vi "Special Folder Path.vi"(8 "error in (no error)":errorcluster, 11 "Special Folder":T1) -> (0 "error out":errorcluster, 3 "Path":path)   [LabVIEW 2013]
doc: "Return the path of the specified special folder. Calls SHGetFolderPathA routine in shell32.dll to determine the answer.\n\nFreeware from Moore Good Ideas, www.mooregoodideas.com. Do not remove this line."
uses:
  Special Folder Enum.ctl
  shell32.dll
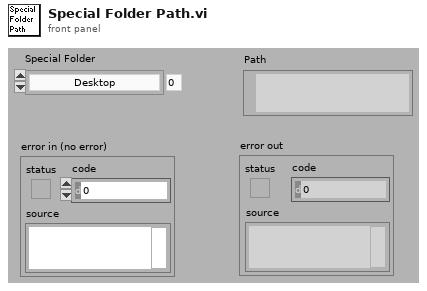
[diagram p1: front panel]
types:
  T1 = typedef "Special Folder Enum.ctl" = enum32{"Desktop", "Err<Internet>", "Programs", "Err<Controls>", "Err<Printers>", "Personal (MyDocuments)", "Favorites", "Startup", "Recent", "SendTo", "Err<RecycleBin>", "StartMenu", "Err<MyDocuments>", "MyMusic", "MyVideo", "Err<0x000F>", "DesktopDirectory", "Err<Drives>", "Err<Network>", "NetHood", "Fonts", "Templates", "CommonStartMenu", "CommonPrograms", "CommonStartup", "CommonDesktopDirectory", "AppData", "PrintHood", "LocalAppData", "Err<AltStartup>", "Err<CommonAltStartup>", "CommonFavorites", "InternetCache", "Cookies", "History", "CommonAppData", "Windows", "System", "ProgramFiles", "MyPictures", "Profile", "System32", "Err<0x002A>", "ProgramFilesCommon", "Err<0x002C>", "CommonTemplates", "CommonDocuments", "CommonAdminTools", "AdminTools"}
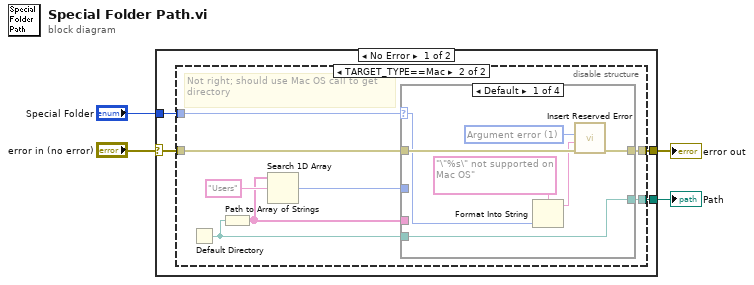
[diagram p0: block diagram]
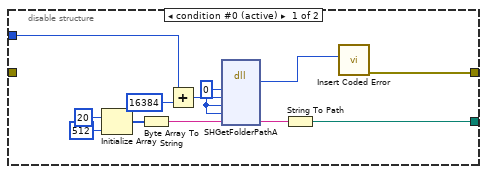
[diagram p2: hidden frame]
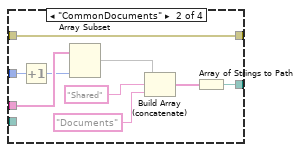
[diagram p3: hidden frame]
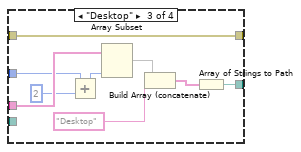
[diagram p4: hidden frame]
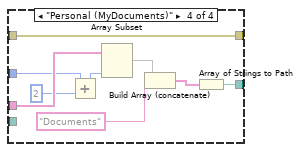
[diagram p5: hidden frame]
diagram:
  n1 = case shown="No Error" "error in (no error)" {
    selector: "error in (no error)" -> [w5 w63]
    tunnel: [w8 w63] -> w4
    tunnel: [w7 _] -> w2
    tunnel: "Special Folder" -> [w6 _]
    frame No Error {
      n2 = disable-structure shown="TARGET_TYPE==Mac" {
        disable-tunnel: [w13 w23] -> w8
        disable-tunnel: [w10 w25] -> w7
        disable-tunnel: w6 -> [w9 w28]
        disable-tunnel: w5 -> [_ w26]
        frame condition #0 (active) {
          w20 = 0 ("hwndOwner")
          n3 = Initialize Array(u8 20 ("element"), 512 ("dimension size")) -> (w17:u8[])
          n4 = Byte Array To String(unsigned byte array=w17) -> (string=w16:string)
          n5 = Add(x=w9, y=u32 16384 ("nFolder")) -> (x+y=w14:u32)
          n6 = dll-call lib="shell32.dll" fn="SHGetFolderPathA"("hwndOwner"=w20, "nFolder"=w14, "hToken"=w20, "dwFlags"=w20, "pszPath"=w16) -> ("HRESULT"=w11:i32, "pszPath"=w12:string)  [unwired: 7 in, 2 out]
          n7 = String To Path(string=w12) -> (path=w10:path)
          n8 = call "Insert Coded Error.vi"("Reserved Error Code"=w11) -> ("error out"=w13:errorcluster)  [unwired: 6 in]
        }
        frame condition #1 {
          # "Not right; should use Mac OS call to get directory"
          n9 = Default Directory() -> (w24:path)
          n10 = Path to Array of Strings(0:w24) -> (2:w21:string[])  [unwired: 1 out]
          n11 = Search 1D Array(1D array=w21, element="Users") -> (index of element=w22:i32)  [unwired: 1 in]
          n12 = case shown="Default" w28 {
            selector: w28 -> [w30 _ _ _]
            tunnel: w26 -> [w33 w43 w52 w61]
            tunnel: [w35 w44 w53 w62] -> w25
            tunnel: w24 -> [w35 _ _ _]
            tunnel: [w34 w43 w52 w61] -> w23
            tunnel: w22 -> [_ w41 w47 w56]
            tunnel: w21 -> [_ w42 w51 w60]
            frame Default {
              w31 = u16 1 items=["No error", "Argument error", "Memory is full", "Out of zone", "End of file", "File already open", "Generic file I/O error", "File not found", "File permission error", "Disk is full", "Duplicate path", "Too many files open", "System feature not enabled", "Resource file not found", "Cannot add resource", "Resource not found", "Image not found", "Image memory error", "Pen does not exist", "Config type invalid", "Config token not found", "Config parse error", "Config memory error", "Bad external code format", "Bad external code offset", "External code not present", "Null window", "Destroy window error", "Null menu", "Print aborted", "Bad print record", "Print driver error", "Windows error during printing", "Memory error during printing", "Print dialog error", "Generic print error", "Invalid device refnum", "Device not found", "Device parameter error", "Device unit error", "Cannot open device", "Device call aborted", "Generic error", "Cancelled by user", "Object ID too low", "Object ID too high", "Object not in heap", "Unknown heap", "Unknown object (invalid DefProc)", "Unknown object (DefProc not in table)", "Message out of range", "Invalid (null) method", "Unknown message", "Manager call not supported", "Bad address", "Network operation in progress", "Network operation timed out", "Connection is busy", "Network attribute not supported", "Network error", "Address in use", "System out of memory", "Connection aborted", "Connection refused", "Not connected", "Already connected", "Connection closed", "Initialization error (interapplication manager)", "Bad occurrence", "Wait on unbound occurrence handler", "Occurrence queue overflow", "Datalog type conflict", "Unused", "Unrecognized type (interapplication manager)", "Memory corrupt", "Failed to make temporary DLL", "Old CIN version", "Drag socket not found", "Failed to load drop-object", "Failed to register OLE object", "Failed to release OLE object", "Format specifier type mismatch", "Unknown format specifier", "Too few format specifiers", "Too many format specifiers", "Scan failed", "Newer CIN version", "OLE Convert", "Runtime menu error", "Password tampered", "Unknown error code"] ("Reserved Error Code (Generic error)")
              n13 = Format Into String(format string="\"%s\" not supported on Mac OS", w30) -> (resulting string=w32:string)  [unwired: 2 in, 1 out]
              n14 = call "Insert Reserved Error.vi"("error in (no error)"=w33, "error description"=w32, "Reserved Error Code (Generic error)"=w31) -> ("error out"=w34:errorcluster)  [unwired: 4 in]
            }
            frame "CommonDocuments" {
              n15 = Increment(x=w41) -> (x+1=w40:i32)
              n16 = Array Subset(array=w42, length=w40) -> (w39:string[])  [unwired: 1 in]
              n17 = Build Array (concatenate)(w39, "Shared" ("element"), "Documents" ("element")) -> (w36:string[])
              n18 = Array of Strings to Path(0:w36) -> (2:w44:path)  [unwired: 1 in]
            }
            frame "Desktop" {
              n19 = Add(x=w47, y=2) -> (x+y=w46:i32)
              n20 = Array Subset(array=w51, length=w46) -> (w50:string[])  [unwired: 1 in]
              n21 = Build Array (concatenate)(w50, "Desktop" ("element")) -> (w48:string[])
              n22 = Array of Strings to Path(0:w48) -> (2:w53:path)  [unwired: 1 in]
            }
            frame "Personal (MyDocuments)" {
              n23 = Add(x=w56, y=2) -> (x+y=w55:i32)
              n24 = Array Subset(array=w60, length=w55) -> (w59:string[])  [unwired: 1 in]
              n25 = Build Array (concatenate)(w59, "Documents" ("element")) -> (w57:string[])
              n26 = Array of Strings to Path(0:w57) -> (2:w62:path)  [unwired: 1 in]
            }
          }
        }
      }
    }
    frame Error {
    }
  }
  "error out" <- w4
  "Path" <- w2
